vi "Image to PNG Data URI.vi"(8 "error in (no error)":errorcluster, 11 "Image data":T1) -> (0 "error out":errorcluster, 2 "Empty image?":bool, 3 "Base64 encoded":string)   [LabVIEW 2019]
uses:
  <vilib>/JDP Science/JDP Science Common Utilities/Base64/Base64 Support.lvlib
  <vilib>/picture/picture.llb/imagedata.ctl
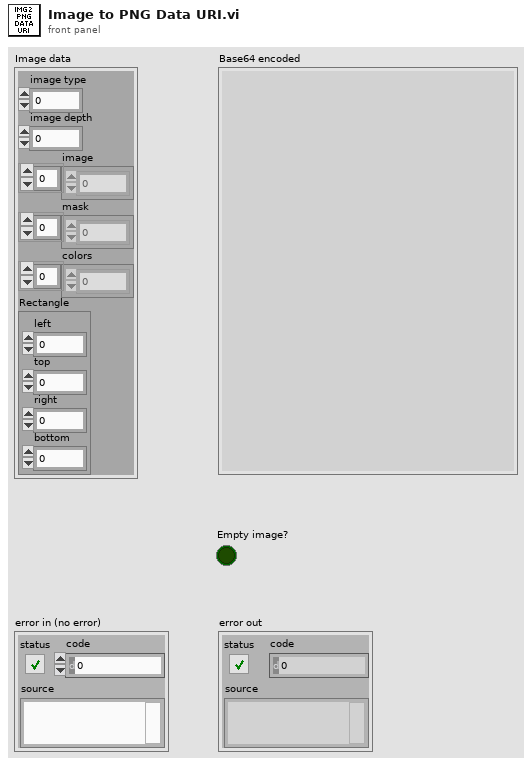
[diagram p1: front panel]
types:
  T1 = typedef "imagedata.ctl" = cluster{"image type":i32, "image depth":i32, "image":u8[], "mask":u8[], "colors":u32[], "Rectangle":cluster{"left":i16, "top":i16, "right":i16, "bottom":i16}}
  T2 = cluster{"left":i16, "top":i16, "right":i16, "bottom":i16}
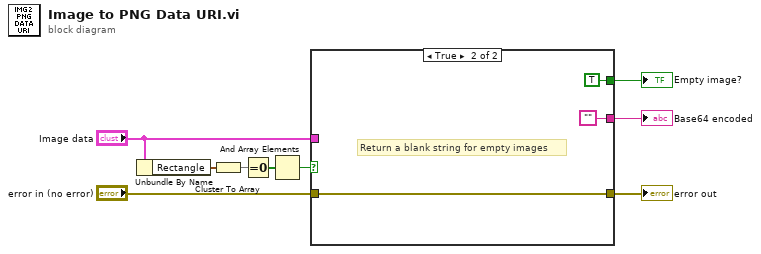
[diagram p0: block diagram]
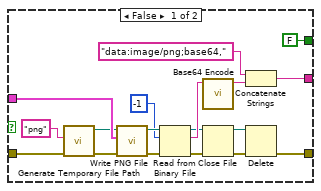
[diagram p2: hidden frame]
diagram:
  n1 = Unbundle By Name("Image data") -> ("Rectangle"=w4:T2)
  n2 = Cluster To Array(cluster=w4) -> (array=w3:i16[])
  n3 = Equal To 0?(x=w3) -> (x = 0?=w2:bool[])
  n4 = And Array Elements(Boolean array=w2) -> (logical AND=w1:bool)
  n5 = case shown="True" w1 {
    tunnel: "Image data" -> [w27 _]
    tunnel: "error in (no error)" -> [w24 w29]
    tunnel: [w19 w29] -> w8
    tunnel: [w13 ""] -> w7
    tunnel: [FALSE ("Empty image?") TRUE ("Empty image?")] -> w5
    frame False {
      n6 = call <vilib>:"Generate Temporary File Path.vi"("error in (no error)"=w24, "Temporary File Extension (tmp)"="png") -> ("error out"=w25:errorcluster, "Unique Temporary File Path"=w26:path)  [unwired: 8 in]
      n7 = call <vilib>:"Write PNG File.vi"("error in (no error)"=w25, "image data"=w27, "path to PNG file"=w26) -> ("error out"=w21:errorcluster, "path"=w20:path)  [unwired: 7 in]
      n8 = Read from Binary File(8:w21, 10:-1 ("count (1)"), 11:w20) -> (0:w18:errorcluster, 2:w22:string, 3:w16:refnum<file>)  [unwired: 3 in, 1 out]
      n9 = call <vilib>:"Base64 Encode.vi"("String to Encode"=w22) -> ("Base64 Encoded"=w12:string)  [unwired: 10 in]
      n10 = Close File(refnum=w16, error in=w18) -> (path=w15:path, error out=w17:errorcluster)
      n11 = Concatenate Strings("data:image/png;base64," ("string"), w12) -> (w13:string)
      n12 = Delete(path (use dialog)=w15, error in=w17) -> (error out=w19:errorcluster)  [unwired: 3 in, 2 out]
    }
    frame True {
      # "Return a blank string for empty images"
    }
  }
  "error out" <- w8
  "Base64 encoded" <- w7
  "Empty image?" <- w5
